vi "ExReprogExample.vi"() -> ()   [LabVIEW 2010]
panel:
  in  "Close Windows":bool
  out "error out":errorcluster
  in  "error in (no error)":errorcluster
  in  "Exposure":dbl format="%.2f"
  # "ExReprogExample:\nDescription: This example shows how to \nreprogram the camera without leaving the\nusers program. This example collects a full\nimage, binned by 2 image, the 4 corners of\nthe CCD."
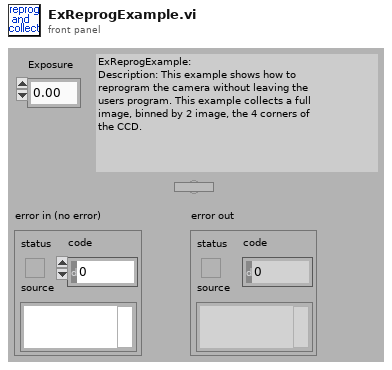
[diagram p1: front panel]
types:
  T1 = cluster{u32, "Xdim":u32, u32, u32, "Ydim":u32, u32}
  T2 = cluster{i32, "Xdim":u32, i32, i32, "Ydim":u32, i32}
  T3 = cluster{u32, "Xdim":u32, i32, u32, "Ydim":u32, i32}
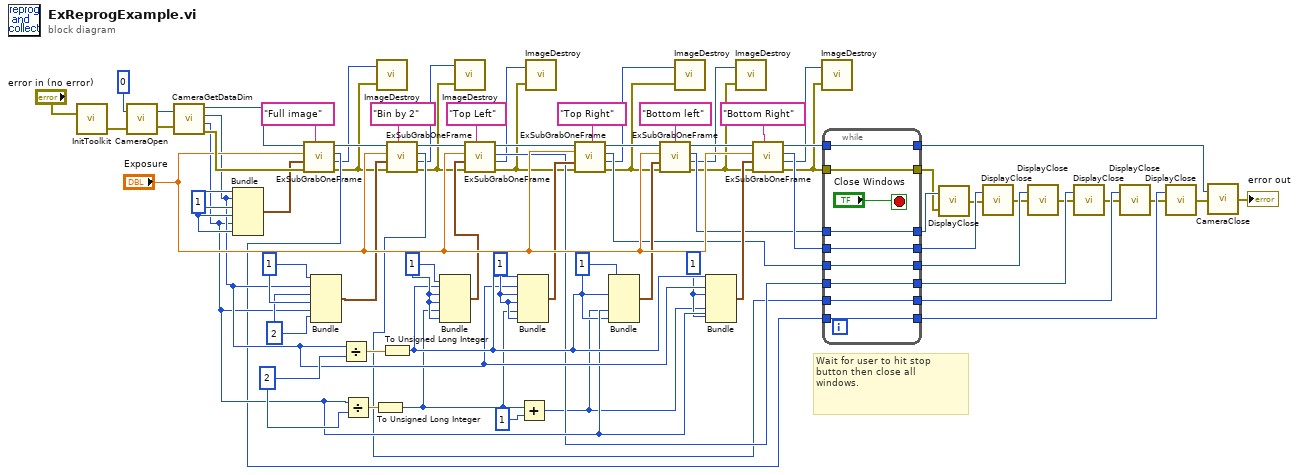
[diagram p0: block diagram]
diagram:
  w39 = 1
  w40 = 1
  w45 = 1
  w47 = 1
  w50 = 2
  w53 = 2
  w54 = 1
  w67 = u32 1
  # "Wait for user to hit stop\nbutton then close all \nwindows."
  n1 = call <userlib>:"InitToolkit.vi"("error in"="error in (no error)") -> ("error out"=w74:errorcluster)
  n2 = call <userlib>:"CameraOpen.vi"("error in"=w74, "Camera Device ID"=0) -> ("error out"=w71:errorcluster, "Camera Handle"=w72:u32)
  n3 = call <userlib>:"CameraGetDataDim.vi"("Camera Handle"=w72, "error in"=w71) -> ("Camera Handle"=w68:u32, "Xdim"=w42:u32, "Ydim"=w41:u32, "error out"=w70:errorcluster)
  n4 = Bundle(w67, "Xdim"=w42, w67, w67, "Ydim"=w41, w67) -> (w66:T1)  [unwired: 1 in]
  n5 = call "ExSubGrabOneFrame.vi"("Display Title"="Full image", "error in"=w70, "ROI Cluster"=w66, "Exposure"="Exposure", "Camera Handle"=w68) -> ("error out"=w14:errorcluster, "Image Handle"=w15:u32, "Display Handle"=w31:u32, "Camera Handle out"=w61:u32)
  n6 = Bundle(w54, "Xdim"=w42, w53, w54, "Ydim"=w41, w53) -> (w52:T2)  [unwired: 1 in]
  n7 = Divide(x=w42, y=w50) -> (x/y=w48:dbl)
  n8 = Divide(x=w41, y=w50) -> (x/y=w49:dbl)
  n9 = To Unsigned Long Integer(number=w49) -> (unsigned 32bit integer=w3:u32)
  n10 = call <userlib>:"ImageDestroy.vi"("error in"=w14, "Data handle"=w15) -> ()  [unwired: 1 out]
  n11 = To Unsigned Long Integer(number=w48) -> (unsigned 32bit integer=w43:u32)
  n12 = call "ExSubGrabOneFrame.vi"("Display Title"="Bin by 2", "error in"=w14, "ROI Cluster"=w52, "Exposure"="Exposure", "Camera Handle"=w61) -> ("error out"=w12:errorcluster, "Image Handle"=w13:u32, "Display Handle"=w32:u32, "Camera Handle out"=w62:u32)
  n13 = Bundle(w47, w43, w47, w47, w3, w47) -> (w46:cluster{i32, u32, i32, i32, u32, i32})  [unwired: 1 in]
  n14 = call <userlib>:"ImageDestroy.vi"("error in"=w12, "Data handle"=w13) -> ()  [unwired: 1 out]
  n15 = call "ExSubGrabOneFrame.vi"("Display Title"="Top Left", "error in"=w12, "ROI Cluster"=w46, "Exposure"="Exposure", "Camera Handle"=w62) -> ("error out"=w11:errorcluster, "Image Handle"=w10:u32, "Display Handle"=w33:u32, "Camera Handle out"=w63:u32)
  n16 = Bundle(w43, "Xdim"=w42, w45, w45, w3, w45) -> (w44:cluster{u32, "Xdim":u32, i32, i32, u32, i32})  [unwired: 1 in]
  n17 = Add(x=w3, y=1) -> (x+y=w1:u32)
  n18 = call <userlib>:"ImageDestroy.vi"("error in"=w11, "Data handle"=w10) -> ()  [unwired: 1 out]
  n19 = call "ExSubGrabOneFrame.vi"("Display Title"="Top Right", "error in"=w11, "ROI Cluster"=w44, "Exposure"="Exposure", "Camera Handle"=w63) -> ("error out"=w9:errorcluster, "Image Handle"=w8:u32, "Display Handle"=w34:u32, "Camera Handle out"=w64:u32)
  n20 = Bundle(w40, w43, w40, w1, "Ydim"=w41, w40) -> (w38:cluster{i32, u32, i32, u32, "Ydim":u32, i32})  [unwired: 1 in]
  n21 = call "ExSubGrabOneFrame.vi"("Display Title"="Bottom left", "error in"=w9, "ROI Cluster"=w38, "Exposure"="Exposure", "Camera Handle"=w64) -> ("error out"=w6:errorcluster, "Image Handle"=w7:u32, "Display Handle"=w35:u32, "Camera Handle out"=w65:u32)
  n22 = call <userlib>:"ImageDestroy.vi"("error in"=w9, "Data handle"=w8) -> ()  [unwired: 1 out]
  n23 = Bundle(w43, "Xdim"=w42, w39, w1, "Ydim"=w41, w39) -> (w37:T3)  [unwired: 1 in]
  n24 = call <userlib>:"ImageDestroy.vi"("error in"=w6, "Data handle"=w7) -> ()  [unwired: 1 out]
  n25 = call "ExSubGrabOneFrame.vi"("Display Title"="Bottom Right", "error in"=w6, "ROI Cluster"=w37, "Exposure"="Exposure", "Camera Handle"=w65) -> ("error out"=w5:errorcluster, "Image Handle"=w4:u32, "Display Handle"=w36:u32, "Camera Handle out"=w51:u32)
  n26 = call <userlib>:"ImageDestroy.vi"("error in"=w5, "Data handle"=w4) -> ()  [unwired: 1 out]
  n27 = while {
    tunnel: w5 -> [w83]
    tunnel: [w83] -> w19
    tunnel: w51 -> [w82]
    tunnel: [w82] -> w18
    tunnel: w36 -> [w80]
    tunnel: w35 -> [w81]
    tunnel: w34 -> [w79]
    tunnel: w33 -> [w78]
    tunnel: w32 -> [w76]
    tunnel: w31 -> [w77]
    tunnel: [w81] -> w30
    tunnel: [w80] -> w29
    tunnel: [w79] -> w28
    tunnel: [w78] -> w27
    tunnel: [w77] -> w25
    tunnel: [w76] -> w26
    stop <- "Close Windows" stop-if-true
  }
  n28 = call <userlib>:"DisplayClose.vi"("error in"=w19, "Display Handle"=w30) -> ("error out"=w24:errorcluster)
  n29 = call <userlib>:"DisplayClose.vi"("error in"=w24, "Display Handle"=w29) -> ("error out"=w23:errorcluster)
  n30 = call <userlib>:"DisplayClose.vi"("error in"=w23, "Display Handle"=w28) -> ("error out"=w22:errorcluster)
  n31 = call <userlib>:"DisplayClose.vi"("error in"=w22, "Display Handle"=w27) -> ("error out"=w21:errorcluster)
  n32 = call <userlib>:"DisplayClose.vi"("error in"=w21, "Display Handle"=w26) -> ("error out"=w20:errorcluster)
  n33 = call <userlib>:"DisplayClose.vi"("error in"=w20, "Display Handle"=w25) -> ("error out"=w17:errorcluster)
  n34 = call <userlib>:"CameraClose.vi"("error in"=w17, "Camera Handle"=w18) -> ("error out"=→"error out":errorcluster)
